vi "Finalize View Init.vi"(8 "error in (no error)":errorcluster, 10 "View Name":string, 11 "Example Controller Actor in":refnum<class "Example Controller Actor.lvclass">) -> (0 "error out":errorcluster, 3 "Example Controller Actor out":refnum<class "Example Controller Actor.lvclass">)   [LabVIEW 2023, in "Example Controller Actor.lvlib" / "Example Controller Actor.lvclass"]
uses:
  Example Controller Actor.lvclass
  C:/Projects/Shared Libraries/Event Actors/Controller Actor/Controller Actor.lvclass
  Example Events/Inited At Event.lvclass
  C:/Projects/Shared Libraries/Event Actors/Event Data Types/Event String/Event String.lvclass
  C:/Projects/Shared Libraries/Event Actors/Event/Event.lvclass
  <vilib>/Utility/error.llb/Error Cluster From Error Code.vi
  <vilib>/ErrorRing/Error Ring.xnode
  Example Controller Actor.lvclass/Example Controller Actor.ctl
  Controller Actor/Controller Actor.lvclass
  C:/Projects/Shared Libraries/Event Actors/Examples/Example Events/Inited At Event.lvclass
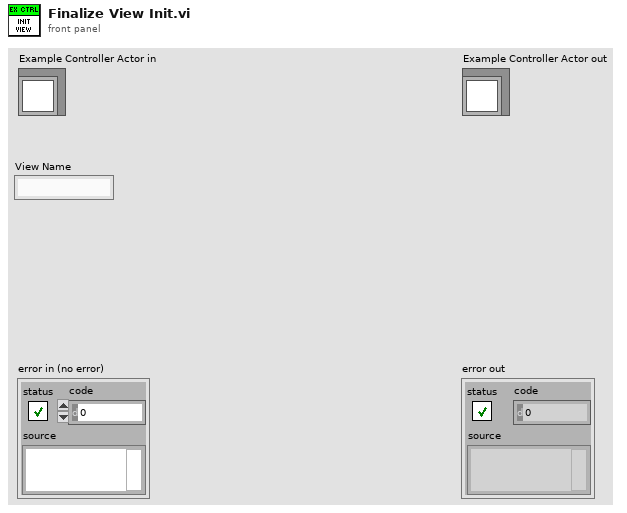
[diagram p1: front panel]
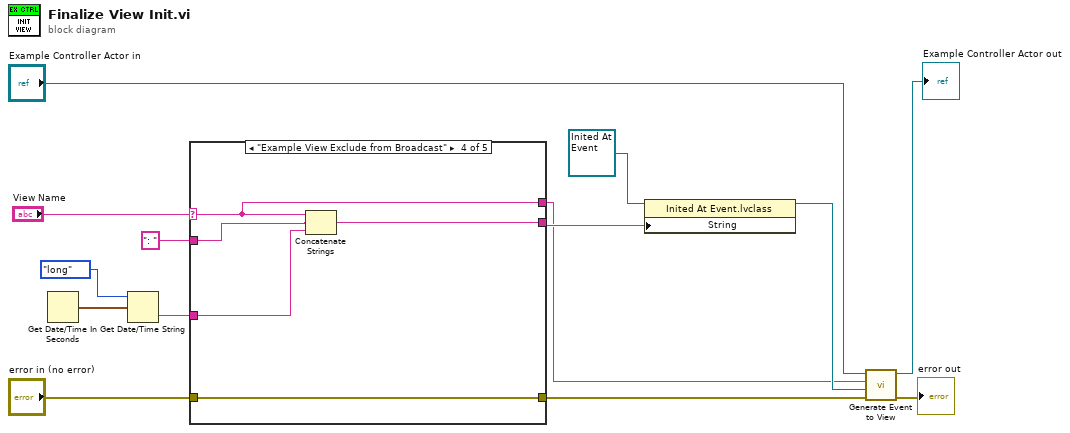
[diagram p0: block diagram]
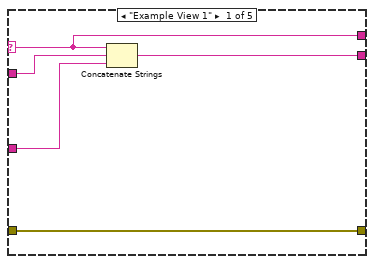
[diagram p2: hidden frame]
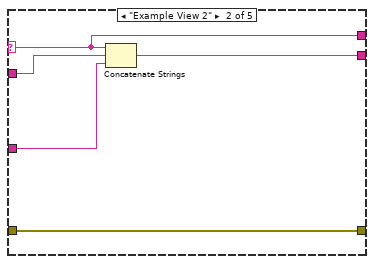
[diagram p3: hidden frame]
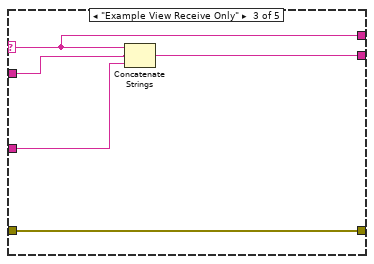
[diagram p4: hidden frame]
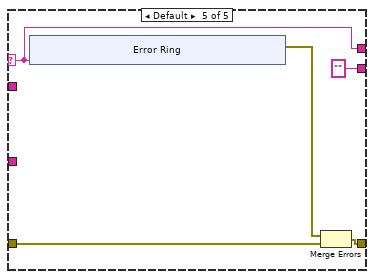
[diagram p5: hidden frame]
diagram:
  n1 = Get Date/Time In Seconds() -> (seconds since 1Jan1904=w13:timestamp)
  n2 = Get Date/Time String(date format (0)=enum16{"short", "long", "abbreviated"}."long", seconds (now)=w13) -> (time string=w11:string)  [unwired: 1 in, 1 out]
  n3 = case shown="\"Example View Exclude from Broadcast\"" "View Name" {
    selector: "View Name" -> [w16 w20 w26 w31 w35]
    tunnel: w11 -> [w19 w24 w29 w34 _]
    tunnel: [w18 w22 w27 w32 ""] -> w5
    tunnel: "error in (no error)" -> [w15 w21 w25 w30 w38]
    tunnel: [w15 w21 w25 w30 w37] -> w7
    tunnel: ": " -> [w17 w23 w28 w33 _]
    tunnel: [w16 w20 w26 w31 w35] -> w3
    frame "Example View 1" {
      n4 = Concatenate Strings(w16, w17, w19) -> (w18:string)
    }
    frame "Example View 2" {
      n5 = Concatenate Strings(w20, w23, w24) -> (w22:string)
    }
    frame "Example View Receive Only" {
      n6 = Concatenate Strings(w26, w28, w29) -> (w27:string)
    }
    frame "Example View Exclude from Broadcast" {
      n7 = Concatenate Strings(w31, w33, w34) -> (w32:string)
    }
    frame Default {
      n8 = xnode "Error Ring"("parameter 0"=w35) -> ("error out"=w39:errorcluster)
      n9 = Merge Errors(w39, w38) -> (w37:errorcluster)
    }
  }
  n10 = property class="Inited At Event.lvclass"(reference=refnum<class "Inited At Event.lvclass"> refnum ("Inited At Event.lvclass"), "String"=w5) -> (reference out=w4:refnum<class "Inited At Event.lvclass">)  [unwired: 1 in, 1 out]
  n11 = call "Generate Event to View.vi"("error in"=w7, "Event"=w4, "View Name"=w3, "Controller Actor In"="Example Controller Actor in") -> ("error out"=→"error out":errorcluster, "Controller Actor Out"=→"Example Controller Actor out":refnum<class "Example Controller Actor.lvclass">)  [unwired: 6 in]
